vi "Client_gen.vi"(9 "Różnica":dbl format="%#_13g", 10 "Time":dbl, 11 "Price":dbl format="%#_13g") -> (3 "Client":T1)   [LabVIEW 2014, in "LukiBrary.lvlib"]
doc: "Przyjmuje czas przyjścia poprzedniego klienta, czas różnicy i kwotę. Zwraca następnego klienta"
uses:
  LukiBrary.lvlib
  Client.ctl
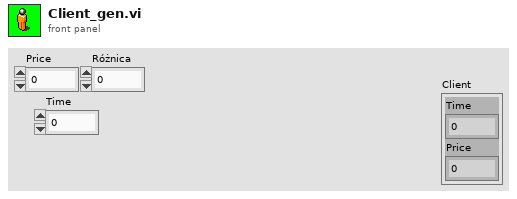
[diagram p1: front panel]
types:
  T1 = typedef "LukiBrary.lvlib/Client.ctl" = cluster{"Time":i32, "Price":i32}
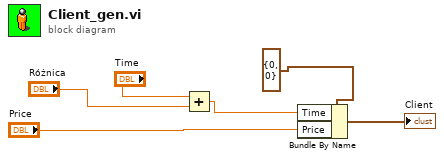
[diagram p0: block diagram]
diagram:
  n1 = Add(x="Time", y="Różnica") -> (x+y=w5:dbl)
  n2 = Bundle By Name(cluster=T1 {"Time"=0, "Price"=0} ("Client"), "Time"=w5, "Price"="Price") -> (→"Client":T1)
